vi "SimpleStandardArcadeDrive.vi"(8 "error in (no error)":errorcluster, 9 "Y axis value":dbl, 10 "X axis value":dbl, 11 "RobotDriveDevRef In":T1={"DevStatus"={"status"=FALSE, "code"=0, "source"=""}, "Motors[]"=[], "Square Inputs"=FALSE, "Max Output"=1.0, "Isochronous"=FALSE}) -> (0 "error out":errorcluster, 3 "RobotDriveDevRef 2":T1={"DevStatus"={"status"=FALSE, "code"=0, "source"=""}, "Motors[]"=[], "Square Inputs"=FALSE, "Max Output"=1.0, "Isochronous"=FALSE})   [LabVIEW 2011]
uses:
  <vilib>/Rock Robotics/WPI/RobotDrive/WPI_RobotDriveDevRef.ctl
  <vilib>/Rock Robotics/WPI/MotorControl/WPI_MotorControlDeviceRef.ctl
  <vilib>/Rock Robotics/SystemInterfaces/Typedef/FPGA_TypedefDigitalModule.ctl
  <vilib>/Rock Robotics/SystemInterfaces/DIO/FPGA_DIOPWMChannel.ctl
  <vilib>/Rock Robotics/WPI/PWM/WPI_PWMDeadband.ctl
  <vilib>/Rock Robotics/WPI/CAN/Jaguar/SubVIs/WPI_CANJaguar_ControlMode.ctl
  <vilib>/Rock Robotics/WPI/PWM/WPI_PWMTransform_ConPane.ctl
  <vilib>/Rock Robotics/SystemInterfaces/NetworkCommunication/NetComm_UsageReport_ResourceType.ctl
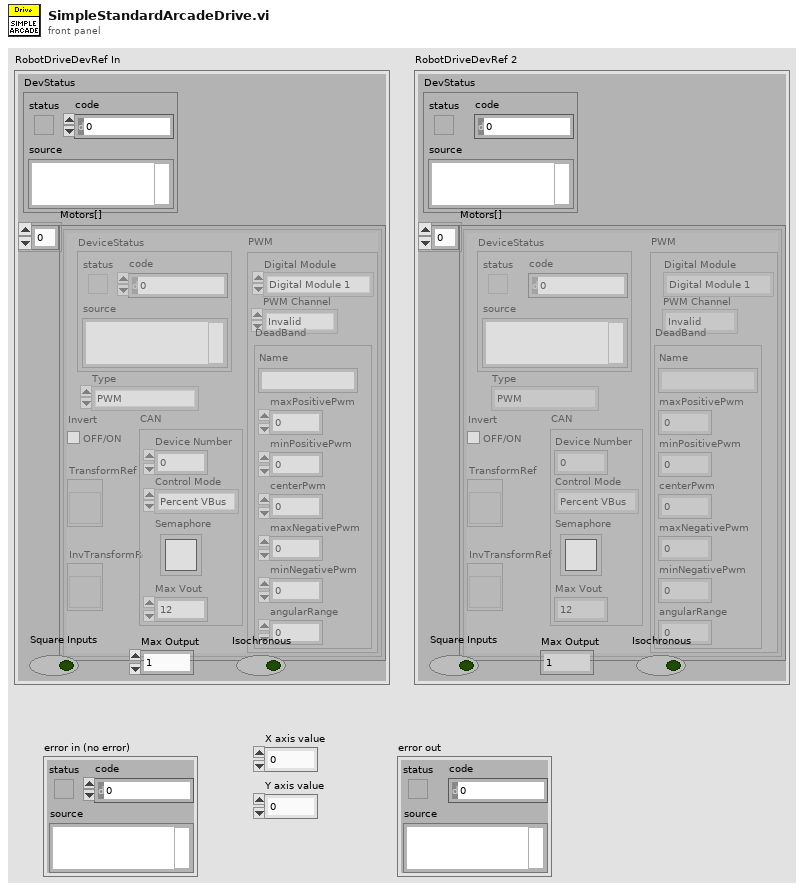
[diagram p1: front panel]
types:
  T1 = typedef "WPI_RobotDriveDevRef.ctl" = cluster{"DevStatus":errorcluster, "Motors[]":T2[], "Square Inputs":bool, "Max Output":dbl, "Isochronous":bool}
  T2 = typedef "WPI_MotorControlDeviceRef.ctl" = cluster{"DeviceStatus":errorcluster, "Type":enum16{"PWM", "CAN"}, "PWM":cluster{"Digital Module":T3, "PWM Channel":T4, "DeadBand":T5}, "CAN":cluster{"Device Number":u8, "Control Mode":T6, "Semaphore":T7, "Max Vout":dbl}, "Invert":bool, "TransformRef":T8, "InvTransformRef":T8}
  T3 = typedef "FPGA_TypedefDigitalModule.ctl" = enum16{"Digital Module 1", "Digital Module 2"}
  T4 = typedef "FPGA_DIOPWMChannel.ctl" = enum8{"PWM 1", "PWM 2", "PWM 3", "PWM 4", "PWM 5", "PWM 6", "PWM 7", "PWM 8", "PWM 9", "PWM 10", "Invalid"}
  T5 = typedef "WPI_PWMDeadband.ctl" = cluster{"Name":string, "maxPositivePwm":i32, "minPositivePwm":i32, "centerPwm":i32, "maxNegativePwm":i32, "minNegativePwm":i32, "angularRange":u16}
  T6 = typedef "WPI_CANJaguar_ControlMode.ctl" = enum8{"Percent VBus", "Current", "Speed", "Position", "Voltage"}
  T7 = typedef "Semaphore RefNum" = refnum<k1>
  T8 = typedef "WPI_PWMTransform_ConPane.ctl" = refnum<vi>
  T9 = typedef "NetComm_UsageReport_ResourceType.ctl" = enum8{"Controller", "Module", "Language", "CANPlugin", "Accelerometer", "ADXL345", "AnalogChannel", "AnalogTrigger", "AnalogTriggerOutput", "CANJaguar", "Compressor", "Counter", "Dashboard", "DigitalInput", "DigitalOutput", "DriverStationCIO", "DriverStationEIO", "DriverStationLCD", "Encoder", "GearTooth", "Gyro", "I2C", "Framework", "Jaguar", "Joystick", "Kinect", "KinectStick", "PIDController", "Preferences", "PWM", "Relay", "RobotDrive", "SerialPort", "Servo", "Solenoid", "SPI", "Task", "Ultrasonic", "Victor", "Button", "Command", "AxisCamera", "PCVideoServer", "SmartDashboard"}
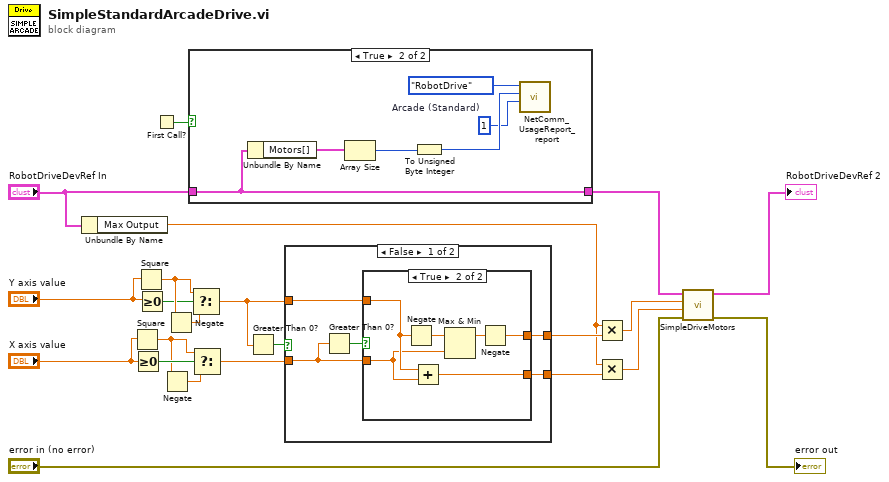
[diagram p0: block diagram]
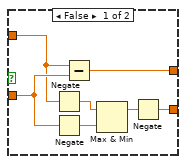
[diagram p3: hidden frame]
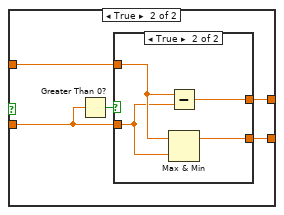
[diagram p4: hidden frame]
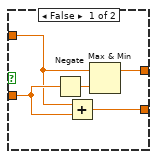
[diagram p5: hidden frame]
diagram:
  n1 = Unbundle By Name("RobotDriveDevRef In") -> ("Max Output"=w15:dbl)
  n2 = Square(x="X axis value") -> (x^2=w12:dbl)
  n3 = Greater Or Equal To 0?(x="X axis value") -> (x >= 0?=w13:bool)
  n4 = Square(x="Y axis value") -> (x^2=w9:dbl)
  n5 = Greater Or Equal To 0?(x="Y axis value") -> (x >= 0?=w8:bool)
  n6 = First Call?() -> (First Call?: T/F=w14:bool)
  n7 = Negate(x=w12) -> (-x=w11:dbl)
  n8 = Negate(x=w9) -> (-x=w10:dbl)
  n9 = case shown="True" w14 {
    tunnel: "RobotDriveDevRef In" -> [w23 w24]
    tunnel: [w23 w24] -> w1
    frame False {
    }
    frame True {
      w27 = u8 1  # Arcade (Standard)
      n10 = Unbundle By Name(w24) -> ("Motors[]"=w26:T2[])
      n11 = Array Size(array=w26) -> (size(s)=w25:i32)
      n12 = To Unsigned Byte Integer(number=w25) -> (unsigned 8bit integer=w28:u8)
      n13 = call <vilib>:"NetComm_UsageReport_report.vi"("Context"=w27, "Instance Number"=w28, "Resource Type"=NetComm_UsageReport_ResourceType."RobotDrive") -> ()  [unwired: 9 in]
    }
  }
  n14 = Select(t=w9, s=w8, f=w10) -> (s? t:f=w21:dbl)
  n15 = Select(t=w12, s=w13, f=w11) -> (s? t:f=w20:dbl)
  n16 = Greater Than 0?(x=w21) -> (x > 0?=w22:bool)
  n17 = case shown="False" w22 {
    tunnel: w20 -> [w33 w51]
    tunnel: w21 -> [w32 w50]
    tunnel: [w31 w49] -> w19
    tunnel: [w30 w48] -> w16
    frame False {
      n18 = Greater Than 0?(x=w33) -> (x > 0?=w34:bool)
      n19 = case shown="True" w34 {
        tunnel: w33 -> [w41 w43]
        tunnel: w32 -> [w39 w44]
        tunnel: [w35 w45] -> w31
        tunnel: [w36 w42] -> w30
        frame False {
          n20 = Negate(x=w39) -> (-x=w40:dbl)
          n21 = Negate(x=w41) -> (-x=w38:dbl)
          n22 = Subtract(x=w39, y=w41) -> (x-y=w35:dbl)
          n23 = Max & Min(x=w40, y=w38) -> (max(x,y)=w37:dbl)  [unwired: 1 out]
          n24 = Negate(x=w37) -> (-x=w36:dbl)
        }
        frame True {
          n25 = Negate(x=w44) -> (-x=w47:dbl)
          n26 = Add(x=w44, y=w43) -> (x+y=w42:dbl)
          n27 = Max & Min(x=w47, y=w43) -> (max(x,y)=w46:dbl)  [unwired: 1 out]
          n28 = Negate(x=w46) -> (-x=w45:dbl)
        }
      }
    }
    frame True {
      n29 = Greater Than 0?(x=w51) -> (x > 0?=w52:bool)
      n30 = case shown="True" w52 {
        tunnel: w51 -> [w57 w59]
        tunnel: w50 -> [w54 w60]
        tunnel: [w55 w58] -> w49
        tunnel: [w53 w61] -> w48
        frame False {
          n31 = Negate(x=w57) -> (-x=w56:dbl)
          n32 = Add(x=w54, y=w57) -> (x+y=w53:dbl)
          n33 = Max & Min(x=w54, y=w56) -> (max(x,y)=w55:dbl)  [unwired: 1 out]
        }
        frame True {
          n34 = Subtract(x=w60, y=w59) -> (x-y=w58:dbl)
          n35 = Max & Min(x=w60, y=w59) -> (max(x,y)=w61:dbl)  [unwired: 1 out]
        }
      }
    }
  }
  n36 = Multiply(x=w15, y=w19) -> (x*y=w2:dbl)
  n37 = Multiply(x=w15, y=w16) -> (x*y=w3:dbl)
  n38 = call "SimpleDriveMotors.vi"("error in (no error)"="error in (no error)", "RightSpeed"=w3, "LeftSpeed"=w2, "RobotDriveDevRef In"=w1) -> ("error out"=→"error out":errorcluster, "RobotDriveDevRef Out"=→"RobotDriveDevRef 2":T1)  [unwired: 6 in]
